vi "SetWaitValues.vi"(6 "SynchToClk(ms)":i32, 8 "error in (no error)":errorcluster caption="entrée d'erreur (pas d'erreur)", 9 "Afterwait(ms)":u32, 10 "Beforewait(ms)":u32, 11 "BaseDevice en entrée":refnum<class "BaseDevice.lvclass"> caption="DNL_LabVIEW Object in") -> (0 "error out":errorcluster caption="sortie d'erreur", 3 "BaseDevice en sortie":refnum<class "BaseDevice.lvclass"> caption="DNL_LabVIEW Object out")   [LabVIEW 2019, in "BaseDevice.lvclass"]
uses:
  BaseDevice.lvclass
  BaseDevice.lvclass/BaseDevice.ctl
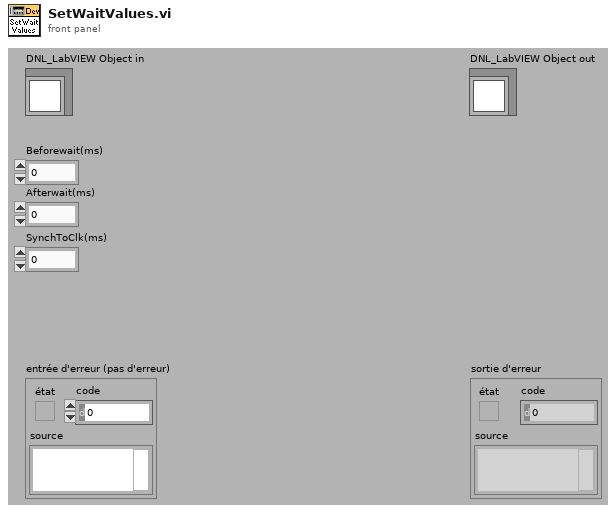
[diagram p1: front panel]
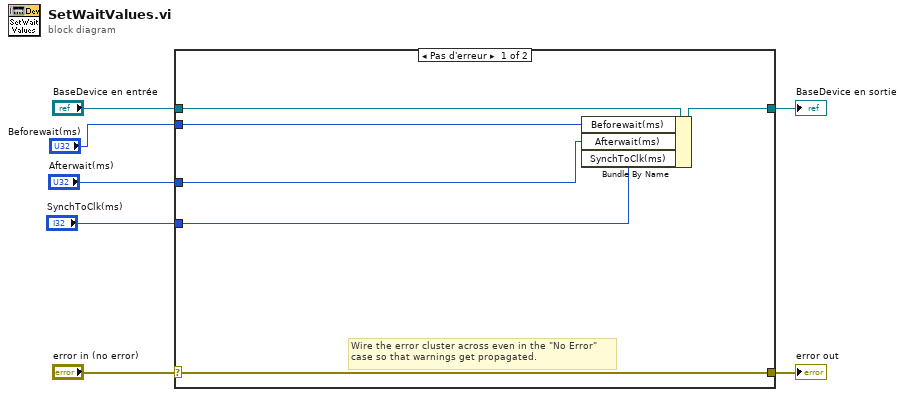
[diagram p0: block diagram]
diagram:
  n1 = case shown="Pas d'erreur" "error in (no error)" {
    selector: "error in (no error)" -> [w13 w15]
    tunnel: [w13 w15] -> w6
    tunnel: [w11 w14] -> w4
    tunnel: "BaseDevice en entrée" -> [w12 w14]
    tunnel: "Beforewait(ms)" -> [w10 _]
    tunnel: "Afterwait(ms)" -> [w9 _]
    tunnel: "SynchToClk(ms)" -> [w8 _]
    frame No Error {
      # "Wire the error cluster across even in the \"No Error\"\ncase so that warnings get propagated."
      n2 = Bundle By Name(cluster=w12, "Beforewait(ms)"=w10, "Afterwait(ms)"=w9, "SynchToClk(ms)"=w8) -> (w11:refnum<class "BaseDevice.lvclass">)
    }
    frame Error {
    }
  }
  "error out" <- w6
  "BaseDevice en sortie" <- w4
